vi "Get Chan Grp.vi"(8 "error in (no error)":errorcluster, 9 "Selected Grp":T1, 11 "Chassis Cfg":refnum<class "ChassisCfg.lvclass">) -> (0 "error out":errorcluster, 3 "Chan Group":refnum<class "ChanGrp.lvclass">)   [LabVIEW 2018, in "Configuration Grandmaster.lvlib" / "ChassisCfg.lvclass"]
uses:
  ChassisCfg.lvclass
  Common/Controls/Selected Group.ctl
  Common/Controls/TE_Designator.ctl
  Class Chan Group/ChanGrp.lvclass
  ChassisCfg.lvclass/ChassisCfg.ctl
  Class Timing Group/TimingGrp.lvclass
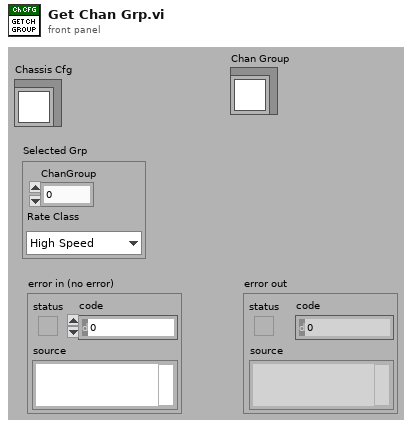
[diagram p1: front panel]
types:
  T1 = typedef "Selected Group.ctl" = cluster{"ChanGroup":i32, "Rate Class":T2}
  T2 = typedef "TE_Designator.ctl" = enum16{"High Speed", "Low Speed"}
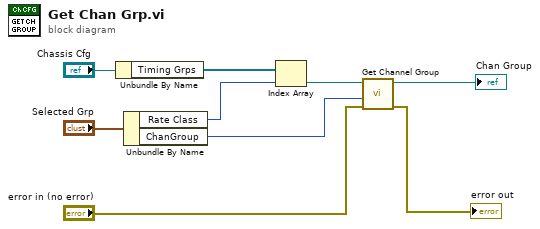
[diagram p0: block diagram]
diagram:
  n1 = Unbundle By Name("Chassis Cfg") -> ("Timing Grps"=w3:refnum<class "TimingGrp.lvclass">[])
  n2 = Unbundle By Name("Selected Grp") -> ("Rate Class"=w2:T2, "ChanGroup"=w8:i32)
  n3 = Index Array(array=w3, index=w2) -> (element=w1:refnum<class "TimingGrp.lvclass">)
  n4 = call "Get Channel Group.vi"("error in (no error)"="error in (no error)", "ChanGroup"=w8, "TimingGrp in"=w1) -> ("error out"=→"error out":errorcluster, "Chan Gropu"=→"Chan Group":refnum<class "ChanGrp.lvclass">)  [unwired: 7 in]
